vi "Get Array Element at Index - String.vi"(8 "error in (no error)":errorcluster, 9 "Default Value":string, 10 "Index":i32, 11 "YAML Parser in":refnum<class "YAML Parser.lvclass">) -> (0 "error out":errorcluster, 1 "Is Null?":bool, 2 "String":string, 3 "YAML Parser out":refnum<class "YAML Parser.lvclass">)   [LabVIEW 2015, in "YAML Parser.lvclass"]
uses:
  YAML Parser.lvclass
  YAML Parser.lvclass/YAML Parser.ctl
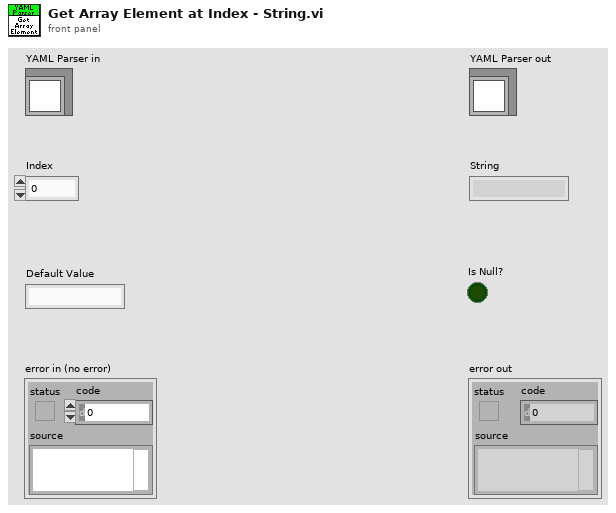
[diagram p1: front panel]
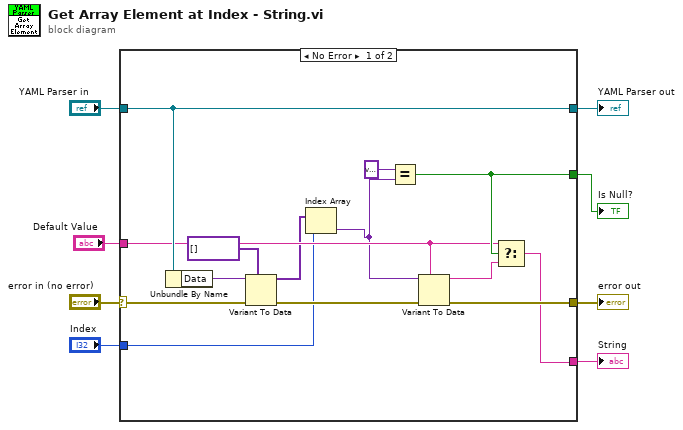
[diagram p0: block diagram]
diagram:
  n1 = case shown="No Error" "error in (no error)" {
    selector: "error in (no error)" -> [w22 w24]
    tunnel: [w19 w24] -> w7
    tunnel: [w21 w23] -> w5
    tunnel: "YAML Parser in" -> [w21 w23]
    tunnel: "Default Value" -> [w16 _]
    tunnel: "Index" -> [w9 _]
    tunnel: [w14 _] -> w2
    tunnel: [w17 _] -> w1
    frame No Error {
      n2 = Unbundle By Name(w21) -> ("Data"=w13:variant)
      n3 = Variant To Data(error in=w22, type=variant[] [], Variant=w13) -> (data=w11:variant[], error out=w20:errorcluster)
      n4 = Index Array(array=w11, index=w9) -> (element=w10:variant)
      n5 = Equal?(x=variant, y=w10) -> (x = y?=w17:bool)
      n6 = Variant To Data(error in=w20, type=w16, Variant=w10) -> (data=w15:string, error out=w19:errorcluster)
      n7 = Select(t=w16, s=w17, f=w15) -> (s? t:f=w14:string)
    }
    frame Error {
    }
  }
  "error out" <- w7
  "YAML Parser out" <- w5
  "String" <- w2
  "Is Null?" <- w1
